vi "MiPS_init.vi"(8 "error in":errorcluster, 9 "Axis Group":string(combo)="GRPZ", 10 "Comms Layer":T1, 11 "VISA in":refnum<visa-resource-name>) -> (0 "error out":errorcluster, 1 "ISOBUS address":T4, 2 "ref_out":T2, 3 "status":bool)   [LabVIEW 2019]
uses:
  Mercury iXX Modules/Public/Controls/ISOBus Address.ctl
  Mercury iXX Modules/Public/Controls/Mercury Reference.ctl
  Mercury iXX Modules/Public/Controls/Comms Transport Layer.ctl
  Mercury iXX Modules/Private/Controls/Query Dynamic Reference.ctl
  Mercury iXX Modules/Public/Controls/Serial Settings.ctl
  Mercury iXX Modules/Public/Libraries/System/Open/Open System.vi
  Mercury iXX Modules/Public/Libraries/System/Read/Catalogue (Read).vi
  Mercury iXX Modules/Public/Libraries/Magnet/Open/Open Magnet Device.vi
  Mercury iXX Modules/Mercury iXX.lvlib
  Mercury iXX Modules/Public/Libraries/System.lvlib
  Mercury iXX Modules/Public/Libraries/Magnet.lvlib
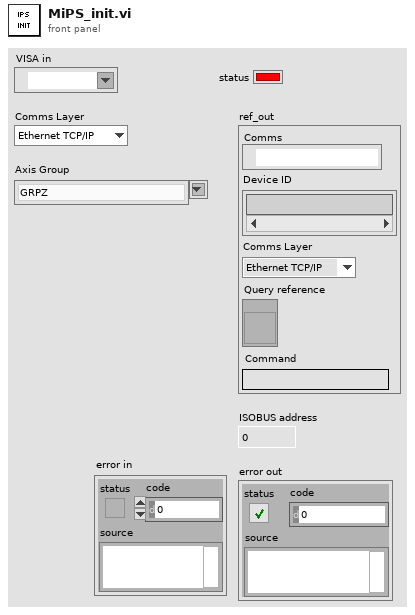
[diagram p1: front panel]
types:
  T1 = typedef "Mercury iXX.lvlib/Comms Transport Layer.ctl" = enum16{"Ethernet TCP/IP", "USB", "ISOBus - RS-232", "GPIB"}
  T2 = typedef "Mercury iXX.lvlib/Mercury Reference.ctl" = cluster{"Comms":refnum<visa-resource-name>, "Device ID":string[], "Comms Layer":T1, "Command":string, "Query reference":T3}
  T3 = typedef "Mercury iXX.lvlib/Query Dynamic Reference.ctl" = refnum<vi>
  T4 = typedef "Mercury iXX.lvlib/ISOBus Address.ctl" = i32
  T5 = typedef "Mercury iXX.lvlib/Serial Settings.ctl" = cluster{"Baud Rate":u32, "Parity":u16, "Data Bits":u16, "Stop Bits":u16, "Flow Control":u16}
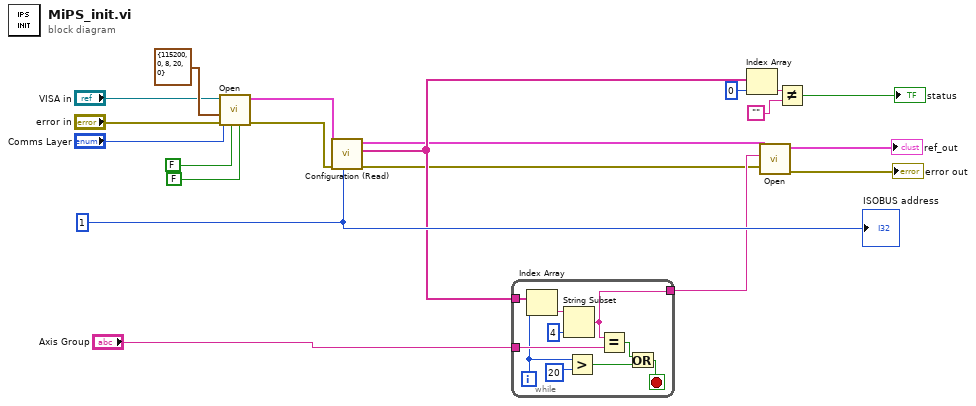
[diagram p0: block diagram]
diagram:
  w19 = T4 1 ("ISOBUS address")
  n1 = call-poly "Open.vi"("Clear Previous Connections (False)"=FALSE, "ID Query (True)"=FALSE, "error in (no error)"="error in", "Serial Configuration"=T5 {"Baud Rate"=115200, "Parity"=0, "Data Bits"=8, "Stop Bits"=20, "Flow Control"=0}, "Comms Layer"="Comms Layer", "VISA resource name"="VISA in") -> ("error out"=w9:errorcluster, "Mercury Reference Out"=w4:T2)  [unwired: 1 in, 3 out]
  n2 = call-poly "Configuration (Read).vi"("ISOBUS address"=w19, "error in"=w9, "Mercury Reference In"=w4) -> ("error out"=w10:errorcluster, "Devices"=w17:string[], "Mercury Reference Out"=w2:T2)  [unwired: 5 in, 1 out]
  n3 = while {
    tunnel: w17 -> [w30]
    tunnel: [w21] -> w18
    tunnel: "Axis Group" -> [w27]
    i -> [w25]
    stop <- w24 stop-if-true
    n4 = Index Array(array=w30, index=w25) -> (element=w28:string)
    n5 = String Subset(string=w28, length (rest)=4 ("length (rest)")) -> (substring=w21:string)  [unwired: 1 out]
    n6 = Greater?(x=w25, y=20) -> (0:w23:bool)
    n7 = Equal?(x=w21, y=w27) -> (x = y?=w22:bool)
    n8 = Or(x=w22, y=w23) -> (x .or. y?=w24:bool)
  }
  n9 = Index Array(array=w17, index=0) -> (element=w7:string)
  n10 = call-poly "Open.vi"("error in (no error)"=w10, "Device Identifier"=w18, "Mercury Reference In"=w2) -> ("error out"=→"error out":errorcluster, "Mercury Reference Out"=→"ref_out":T2)  [unwired: 7 in]
  n11 = Not Equal?(x=w7, y="") -> (x != y?=→"status":bool)
  "ISOBUS address" <- w19
